vi "SMO.UI.ByRefWithEvents.TestLauncher.vi"() -> ()   [LabVIEW 2013, in "SMO.UI.ByRefWithEvents.lvclass"]
doc: "JKI State Machine Objects (SMO) 1.0.0.5\nJKI - JKI\nCopyright (c) 2016, JKI"
uses:
  SMO.UI.ByRefWithEvents.lvclass
  <vilib>/JKI/JKI SMO/SMO/SMO.lvclass
  <vilib>/JKI/JKI SMO/SMO.UI/SMO.UI.lvclass
panel:
  in  "Send":bool
  in  "Data":string
  out "error out":errorcluster
  in  "Stop":bool
  # "SMO UI Test Launcher"
  # "For instructions on how to use the JKI State Machine Objects, examples and video tutorials, visit:\nhttp://jki.net/state-machine-objects/\n\nJKI State Machine Objects™\nhttp://jki.net/state-machine-objects/\nCopyright (C) 2005-2015, JKI <info@jki.net>\nALL RIGHTS RESERVED"
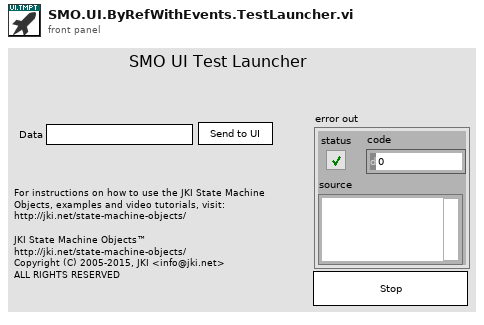
[diagram p1: front panel]
types:
  T1 = cluster{"SMO.Template Public Events":refnum<event-registration>, "SMO.UI Public Events":refnum<event-registration>}
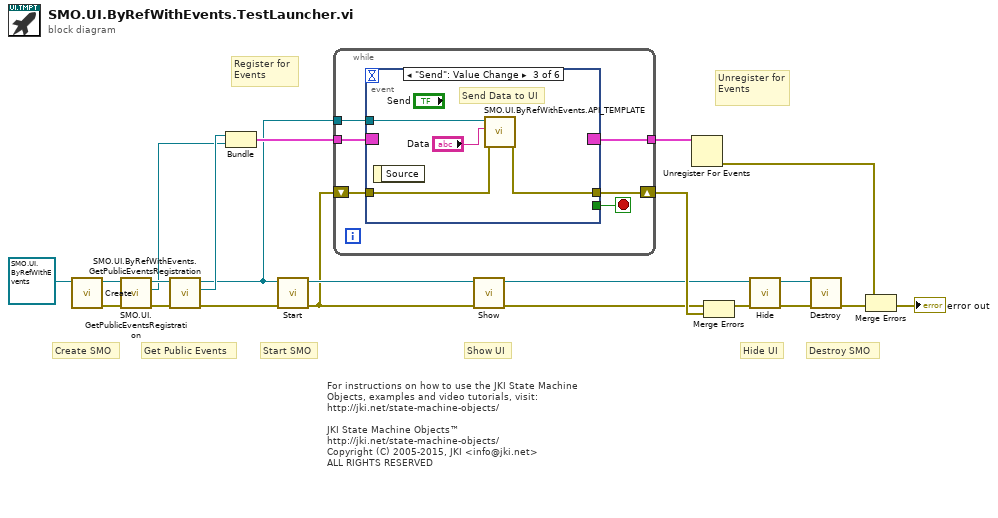
[diagram p0: block diagram]
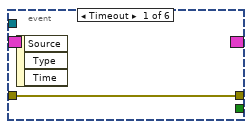
[diagram p2: hidden frame]
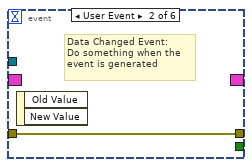
[diagram p3: hidden frame]
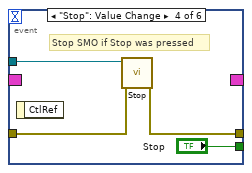
[diagram p4: hidden frame]
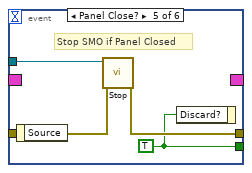
[diagram p5: hidden frame]
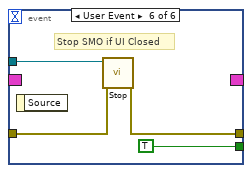
[diagram p6: hidden frame]
diagram:
  # "Hide UI"
  # "Show UI"
  # "For instructions on how to use the JKI State Machine Objects, examples and video tutorials, visit:\nhttp://jki.net/state-machine-objects/\n\nJKI State Machine Objects™\nhttp://jki.net/state-machine-objects/\nCopyright (C) 2005-2015, JKI <info@jki.net>\nALL RIGHTS RESERVED"
  # "Get Public Events"
  # "Start SMO"
  # "Destroy SMO"
  # "Create SMO"
  # "Unregister for Events"
  # "Register for Events"
  n1 = call <vilib>:"Create.vi"("SMO"=refnum<class "SMO.UI.ByRefWithEvents.lvclass"> refnum ("SMO.Template.lvclass")) -> ("error out"=w5:errorcluster, "SMO out"=w3:refnum<class "SMO.UI.ByRefWithEvents.lvclass">)  [unwired: 9 in]
  n2 = call <vilib>:"SMO.UI.GetPublicEventsRegistration.vi"("error in (no error)"=w5, "SMO.UI"=w3) -> ("error out"=w4:errorcluster, "SMO.UI Public Events"=w1:refnum<event-registration>, "SMO.UI out"=w2:refnum<class "SMO.UI.ByRefWithEvents.lvclass">)  [unwired: 7 in]
  n3 = call "SMO.UI.ByRefWithEvents.GetPublicEventsRegistration.vi"("error in (no error)"=w4, "SMO.UI.ByRefWithEvents"=w2) -> ("error out"=w15:errorcluster, "SMO.Template Public Events"=w14:refnum<event-registration>, "SMO.UI.ByRefWithEvents out"=w13:refnum<class "SMO.UI.ByRefWithEvents.lvclass">)  [unwired: 7 in]
  n4 = Bundle("SMO.Template Public Events"=w14, "SMO.UI Public Events"=w1) -> (w21:T1)  [unwired: 1 in]
  n5 = call <vilib>:"Start.vi"("error in (no error)"=w15, "SMO"=w13) -> ("error out"=w11:errorcluster, "SMO out"=w12:refnum<class "SMO.UI.ByRefWithEvents.lvclass">)  [unwired: 8 in]
  n6 = while {
    shift-right: [w27] -> w20
    shift-left: w11 -> [w26]
    tunnel: w21 -> [w25]
    tunnel: [w24] -> w22
    tunnel: w13 -> [w23]
    stop <- w28 stop-if-true
    n7 = event shown="[2] \"Send\": Value Change" {
      selector: w25 -> [_ _ _ _ _ _]
      dyn-events: [_ _ _ _ _ _] -> w24
      timeout: _ -> [_ _ _ _ _ _]
      tunnel: [_ _ _ "Stop" w39 TRUE ("OK")] -> w28
      tunnel: w23 -> [_ _ w34 w36 w42 w46]
      tunnel: [w29 w30 w31 w37 w41 w45] -> w27
      tunnel: w26 -> [w29 w30 w32 w35 w40 w44]
      event Timeout {
        n8 = event-data() -> ()  [unwired: 1 in, 3 out]
      }
      event User Event {
        # "Data Changed Event:\nDo something when the\nevent is generated"
        n9 = event-data() -> ()  [unwired: 1 in, 2 out]
      }
      event "Send": Value Change {
        # "Send Data to UI"
        n10 = event-data() -> ()  [unwired: 1 in, 1 out]
        n11 = call "SMO.UI.ByRefWithEvents.API_TEMPLATE.vi"("error in (no error)"=w32, "myData"="Data", "SMO.UI.ByRefWithEvents"=w34) -> ("error out"=w31:errorcluster)  [unwired: 6 in, 2 out]
      }
      event "Stop": Value Change {
        # "Stop SMO if Stop was pressed"
        n12 = event-data() -> ()  [unwired: 1 in, 1 out]
        n13 = call <vilib>:"Stop.vi"("error in (no error)"=w35, "SMO"=w36) -> ("error out"=w37:errorcluster)  [unwired: 8 in, 1 out]
      }
      event Panel Close? {
        w39 = TRUE ("OK")
        # "Stop SMO if Panel Closed"
        n14 = event-data() -> ()  [unwired: 1 in, 1 out]
        n15 = call <vilib>:"Stop.vi"("error in (no error)"=w40, "SMO"=w42) -> ("error out"=w41:errorcluster)  [unwired: 8 in, 1 out]
        n16 = event-data("Discard?"=w39) -> ()  [unwired: 1 in, 1 out]
      }
      event User Event {
        # "Stop SMO if UI Closed"
        n17 = event-data() -> ()  [unwired: 1 in, 1 out]
        n18 = call <vilib>:"Stop.vi"("error in (no error)"=w44, "SMO"=w46) -> ("error out"=w45:errorcluster)  [unwired: 8 in, 1 out]
      }
    }
  }
  n19 = call <vilib>:"Show.vi"("error in (no error)"=w11, "SMO.UI"=w12) -> ("error out"=w10:errorcluster, "SMO.UI out"=w9:refnum<class "SMO.UI.ByRefWithEvents.lvclass">)  [unwired: 8 in]
  n20 = Unregister For Events(event registration refnum=w22) -> (error out=w19:errorcluster)  [unwired: 1 in]
  n21 = Merge Errors(w10, w20) -> (w7:errorcluster)
  n22 = call <vilib>:"Hide.vi"("error in (no error)"=w7, "SMO.UI"=w9) -> ("error out"=w6:errorcluster, "SMO.UI out"=w8:refnum<class "SMO.UI.ByRefWithEvents.lvclass">)  [unwired: 8 in]
  n23 = call <vilib>:"Destroy.vi"("error in (no error)"=w6, "SMO"=w8) -> ("error out"=w17:errorcluster)  [unwired: 9 in]
  n24 = Merge Errors(w19, w17) -> (→"error out":errorcluster)
